vi "ConfigDialogIterator.vi"(4 "device NO":i8, 5 "CHS":T3 {"display" format="%b"}) -> (0 "CAl":T5, 1 "left cell text":string[](array[string]), 2 "ch":string)   [LabVIEW 2011]
uses:
  signal type.ctl
  gain.ctl
  singlechtype.ctl
  CHS.ctl
panel:
  in  "type":T1
  in  "Gain":T2
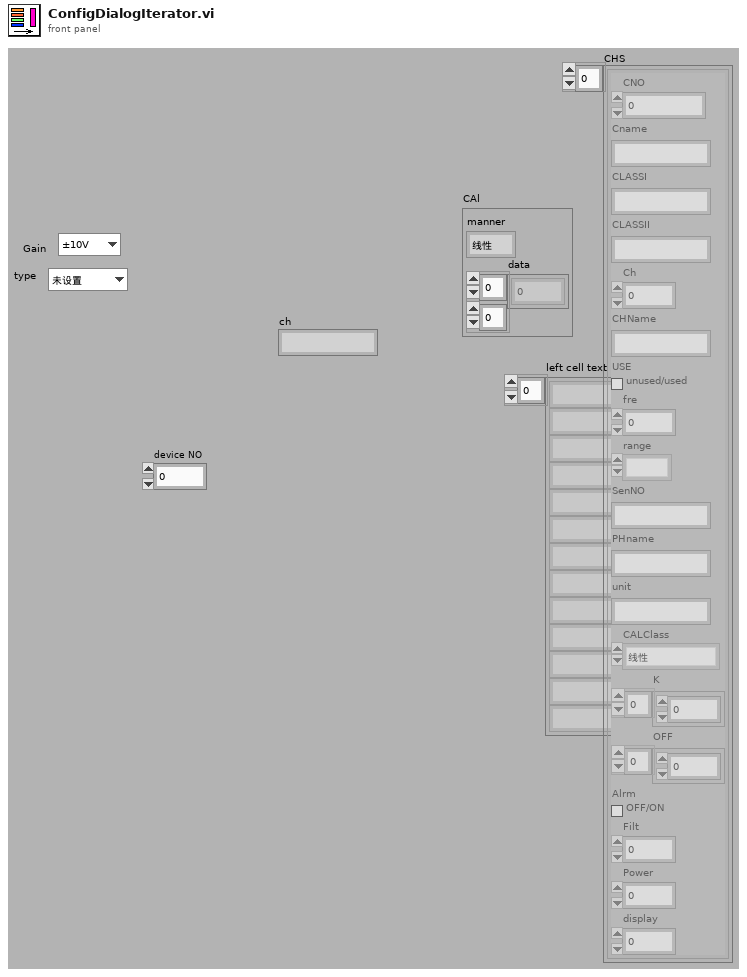
[diagram p1: front panel]
types:
  T1 = typedef "signal type.ctl" = enum16{"未设置", "volet", "current", "vibration", "electric charge ", "resistance "}
  T2 = typedef "gain.ctl" = enum16{"±10V", "±5V", "±2.5V", "±1V", "±500mV", "±100mV", "10V", "5V", "2.5V", "1V", "500mV", "100mV"}
  T3 = typedef "CHS.ctl" = T4[]
  T4 = typedef "singlechtype.ctl" = cluster{"CNO":u8, "Cname":string, "CLASSI":string, "CLASSII":string, "Ch":u8, "CHName":string, "USE":bool, "fre":dbl, "range":enum16{""}, "SenNO":string, "PHname":string, "unit":string, "CALClass":enum8{"线性", "查表", "公式"}, "K":dbl[], "OFF":dbl[], "Alrm":bool, "Filt":dbl, "Power":u8, "display":u8}
  T5 = cluster{"manner":enum16{"线性", "查表"}, "data":dbl[][]}
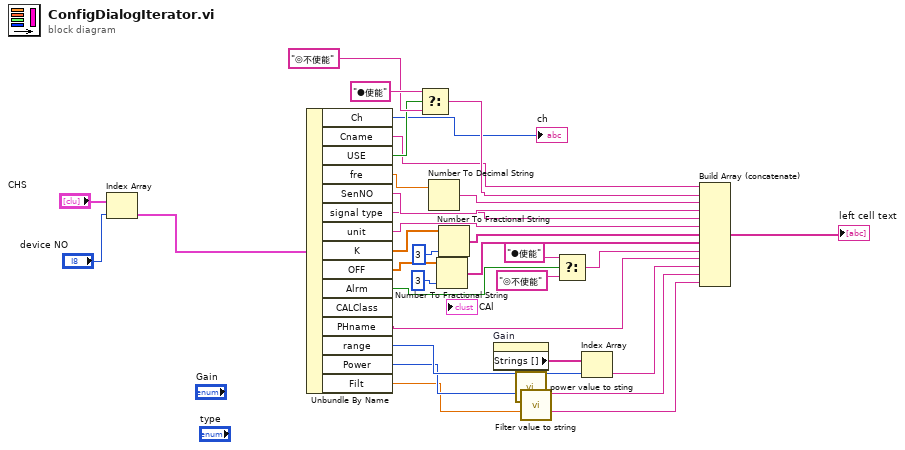
[diagram p0: block diagram]
diagram:
  n1 = Index Array(array="CHS", index="device NO") -> (element=w2:T4)
  n2 = Unbundle By Name(w2) -> ("Ch"=→"ch":u8, "Cname"=w11:string, "USE"=w30:bool, "fre"=w21:dbl, "SenNO"=w19:string, "signal type"=w18:string, "unit"=w17:string, "K"=w22:dbl[], "OFF"=w23:dbl[], "Alrm"=w24:bool, "PHname"=w1:string, "range"=w8:enum16{""}, "Power"=w6:u8, "Filt"=w5:dbl)  [unwired: 1 out]
  n3 = Select(t="●使能", s=w30, f="◎不使能") -> (s? t:f=w29:string)
  n4 = Number To Decimal String(number=w21) -> (decimal integer string=w20:string)  [unwired: 1 out]
  n5 = Number To Fractional String(number=w23, precision (6)=i16 3) -> (F-format string=w15:string[])  [unwired: 2 out]
  n6 = Number To Fractional String(number=w22, precision (6)=i16 3) -> (F-format string=w16:string[])  [unwired: 2 out]
  n7 = property on="Gain" class="Enum (strict)"() -> ("Strings []"=w9:string[])  [unwired: 2 in, 2 out]
  n8 = call "power value to sting.vi"("Power"=w6) -> ("power string"=w4:string)  [unwired: 14 out]
  n9 = call "Filter value to string.vi"("filter set"=w5) -> ("filter string"=w3:string)  [unwired: 14 out]
  n10 = Select(t="●使能", s=w24, f="◎不使能") -> (s? t:f=w14:string)
  n11 = Index Array(array=w9, index=w8) -> (element=w7:string)
  n12 = Build Array (concatenate)(w11, w29, w20, w19, w18, w17, w16, w15, w14, w1, w7, w4, w3) -> (→"left cell text":string[])
